vi "MB MFC Zero Flow.vi"(8 "error in (no error)":errorcluster, 11 "TCP Ref":refnum<k5>) -> (0 "error out":errorcluster, 3 "dup TCP Ref":refnum<k5>)   [LabVIEW 2011]
doc: "This VI sends a signal to Zero an MKS Modbus Mass Flow Controller."
uses:
  EtherNet.lib/Modbus/mb Ethernet.llb/MB Modbus Command.ctl
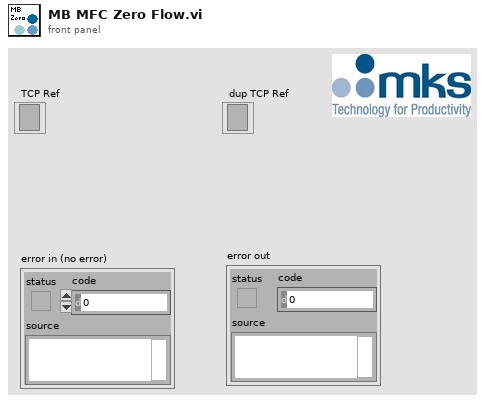
[diagram p1: front panel]
types:
  T1 = typedef "MB Modbus Command.ctl" = cluster{"Function Code":u8, "Starting Address":u16, "Quantity":u16, "Data":u16[], "Discrete":bool[]}
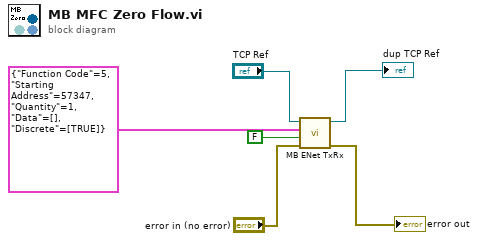
[diagram p0: block diagram]
diagram:
  n1 = call "MB ENet TxRx.vi"("error in (no error)"="error in (no error)", "Use MODBUS Data Unit?"=FALSE, "Modbus Command"=T1 {"Function Code"=5, "Starting Address"=57347, "Quantity"=1, "Data"=[], "Discrete"=[TRUE]}, "TCP Ref:ValBlock"="TCP Ref") -> ("error out"=→"error out":errorcluster, "dup TCP Ref:ValBlock"=→"dup TCP Ref":refnum<k5>)  [unwired: 3 in, 3 out]
